vi "URAPI_Error Dialog.vi"(2 "Error String":string, 3 "Error?":bool, 4 "URAPI Script in":T1) -> (1 "URAPI Script out":T1)   [LabVIEW 2012]
uses:
  <userlib>/BotSpeak/VIs/Direct/URAPI_Control.ctl
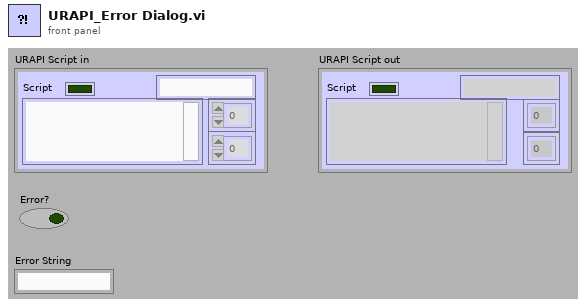
[diagram p1: front panel]
types:
  T1 = typedef "URAPI_Control.ctl" = cluster{"Script":string, "Whiles":u8[], "Ifs":u8[], "Supress Err":bool, "Errors":string}
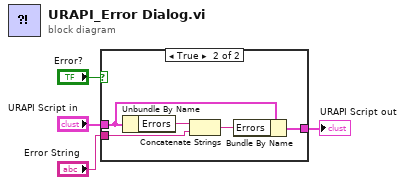
[diagram p0: block diagram]
diagram:
  n1 = case shown="True" "Error?" {
    tunnel: [w5 w10] -> w2
    tunnel: "URAPI Script in" -> [w5 w9]
    tunnel: "Error String" -> [_ w6]
    frame False {
    }
    frame True {
      n2 = Unbundle By Name(w9) -> ("Errors"=w8:string)
      n3 = Concatenate Strings(w8, w6) -> (w7:string)
      n4 = Bundle By Name(cluster=w9, "Errors"=w7) -> (w10:T1)
    }
  }
  "URAPI Script out" <- w2
